vi "MeasurementResultHandling.vi"(8 "error in (no error)":errorcluster, 11 "TestMeasureStep in":refnum<class "TestMeasureStep.lvclass">) -> (0 "error out":errorcluster, 2 "TestStatus":T1, 3 "TestMeasureStep out":refnum<class "TestMeasureStep.lvclass">)   [LabVIEW 2019, in "TestMeasureStep.lvclass"]
uses:
  TestMeasureStep.lvclass
  testSeq/Typedef/TestStatus.ctl
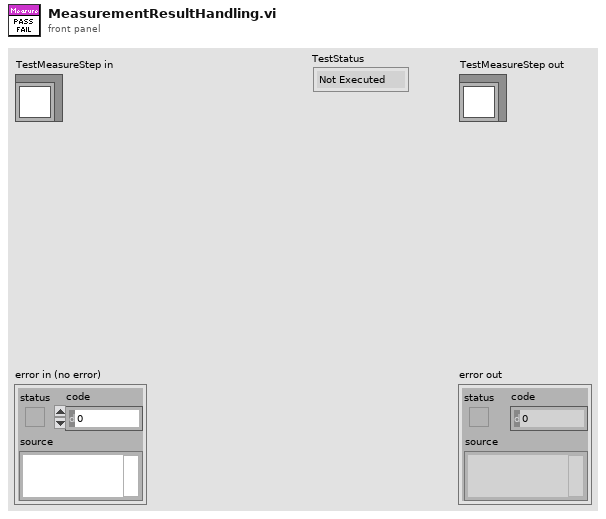
[diagram p1: front panel]
types:
  T1 = typedef "TestStatus.ctl" = enum16{"Not Executed", "Passed", "Failed", "Inconclusive", "Processing"}
  T2 = typedef "TestSeqClass.lvclass/TesstepType.ctl" = cluster{"TestName":string, "Meas":dbl, "Min ":dbl, "Max":dbl, "TestStatus":T1, "StringLimit":string, "StringMeas":string, "Unit":string}
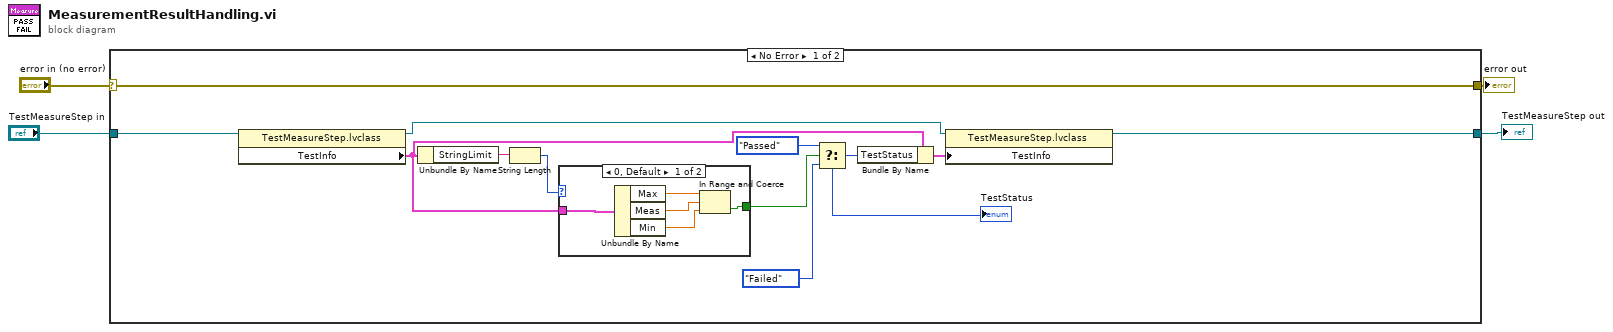
[diagram p0: block diagram]
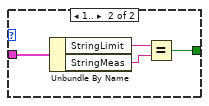
[diagram p2: hidden frame]
diagram:
  n1 = case shown="No Error" "error in (no error)" {
    selector: "error in (no error)" -> [w16 w27]
    tunnel: [w16 w27] -> w3
    tunnel: "TestMeasureStep in" -> [w15 w26]
    tunnel: [w6 w26] -> w1
    frame No Error {
      n2 = property class="TestMeasureStep.lvclass"(reference=w15) -> (reference out=w10:refnum<class "TestMeasureStep.lvclass">, "TestInfo"=w12:T2)  [unwired: 1 in, 1 out]
      n3 = Unbundle By Name(w12) -> ("StringLimit"=w14:string)
      n4 = String Length(string=w14) -> (length=w13:i32)
      n5 = case shown="0, Default" w13 {
        tunnel: w12 -> [w18 w25]
        tunnel: [w17 w22] -> w8
        frame 0, Default {
          n6 = Unbundle By Name(w18) -> ("Max"=w21:dbl, "Meas"=w20:dbl, "Min"=w19:dbl)
          n7 = In Range and Coerce(upper limit=w21, x=w20, lower limit=w19) -> (In Range?=w17:bool)  [unwired: 1 out]
        }
        frame 1.. {
          n8 = Unbundle By Name(w25) -> ("StringLimit"=w24:string, "StringMeas"=w23:string)
          n9 = Equal?(x=w24, y=w23) -> (x = y?=w22:bool)
        }
      }
      n10 = Select(t=TestStatus."Passed" ("TestStatus"), s=w8, f=TestStatus."Failed" ("TestStatus")) -> (s? t:f=w5:T1)
      "TestStatus" <- w5
      n11 = Bundle By Name(cluster=w12, "TestStatus"=w5) -> (w11:T2)
      n12 = property class="TestMeasureStep.lvclass"(reference=w10, "TestInfo"=w11) -> (reference out=w6:refnum<class "TestMeasureStep.lvclass">)  [unwired: 1 in, 1 out]
    }
    frame Error {
    }
  }
  "error out" <- w3
  "TestMeasureStep out" <- w1
